vi "Read Waveform Measurement.vi"(5 "Destination Channel (1: Channel 2)":u16(ring)=1 items=["Channel 1", "Channel 2", "Channel 3", "Channel 4", "MATH", "Reference 1", "Reference 2", "Reference 3", "Reference 4"], 7 "Measurement Function (0: Period)":i32(ring) items=["Period", "Frequency", "Delay", "Rise Time", "Fall Time", "Positive Duty Cycle", "Negative Duty Cycle", "Positive Pulse Width", "Negative Pulse Width", "Burst Width", "Phase", "Positive Overshoot", "Negative Overshoot", "Vpp", "Amplitude", "Voltage High", "Voltage Low", "Voltage Max", "Voltage Min", "Voltage Mean", "Voltage Mean (cycle)", "Voltage RMS", "Voltage RMS (cycle)", "Area", "Cycle Area", "Positive Edge Count", "Negative Edge Count", "Positive Pulse Count", "Negative Pulse Count"], 8 "error in (no error)":errorcluster, 9 "Maximum Time (10000ms)":u32=10000, 10 "Channel (0: Channel 1)":u16(ring) items=["Channel 1", "Channel 2", "Channel 3", "Channel 4", "MATH", "Reference 1", "Reference 2", "Reference 3", "Reference 4"], 11 "VISA resource name":refnum<visa-resource-name>) -> (0 "error out":errorcluster, 2 "Measurement Value":dbl, 3 "VISA resource name out":refnum<visa-resource-name>)   [LabVIEW 2009, in "Tektronix DPO MSO 2000 4000 Series.lvlib"]
doc: "Initiates an acquisition on the channels that you enable with the Configure Channel VI. This VI then waits for the acquisition to complete, obtains a waveform measurement on the channel you specify, and returns the measurement value. The <B>Timeout</B> control specifies the maximum time to wait for operation complete in milliseconds.\n\nNote: You must configure the appropriate reference levels before you call this VI."
uses:
  <instrlib>/Tektronix DPO MSO 2000 4000 Series/Tektronix DPO MSO 2000 4000 Series.lvlib
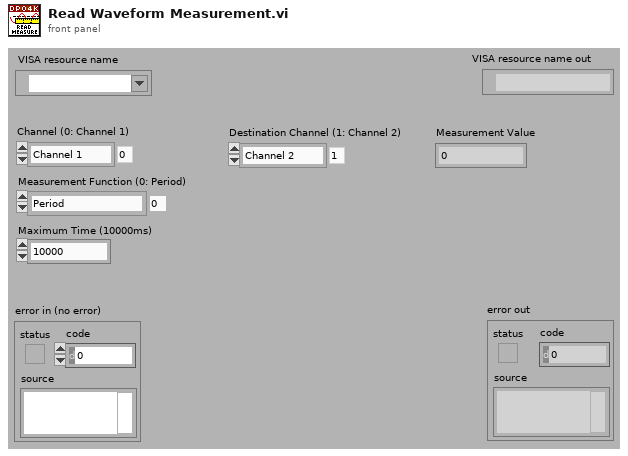
[diagram p1: front panel]
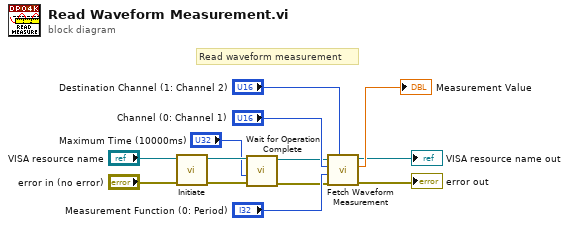
[diagram p0: block diagram]
diagram:
  # "Read waveform measurement"
  n1 = call <instrlib>:"Initiate.vi"("error in (no error)"="error in (no error)", "VISA resource name"="VISA resource name") -> ("error out"=w2:errorcluster, "VISA resource name out"=w3:refnum<visa-resource-name>)  [unwired: 8 in]
  n2 = call <instrlib>:"Wait for Operation Complete.vi"("error in (no error)"=w2, "Maximum Time (10000ms)"="Maximum Time (10000ms)", "VISA resource name"=w3) -> ("error out"=w4:errorcluster, "VISA resource name out"=w5:refnum<visa-resource-name>)  [unwired: 7 in]
  n3 = call <instrlib>:"Fetch Waveform Measurement.vi"("Destination Channel (1: Channel 2)"="Destination Channel (1: Channel 2)", "error in (no error)"=w4, "Measurement Function (0: Period)"="Measurement Function (0: Period)", "Channel (0: Channel 1)"="Channel (0: Channel 1)", "VISA resource name"=w5) -> ("error out"=→"error out":errorcluster, "Measurement Value"=→"Measurement Value":dbl, "VISA resource name out"=→"VISA resource name out":refnum<visa-resource-name>)  [unwired: 4 in]
